vi "FOS_CL_run.vi"() -> ()   [LabVIEW 2019]
uses:
  <vilib>/myRIO/Instrument Drivers/Onboard IO/DIO/typedefs/DIO Reference.ctl
  <vilib>/myRIO/Common/Instrument Driver Framework/Utilities/typedefs/myRIO Generic Hardware Reference.ctl
  <vilib>/myRIO/Common/Instrument Driver Framework/Utilities/typedefs/Hardware Version Enum.ctl
  <vilib>/myRIO/Common/Instrument Driver Framework/Utilities/typedefs/myRIO v1.0 Reference.ctl
  <vilib>/myRIO/Common/Instrument Driver Framework/Utilities/typedefs/Generic FPGA Reference.ctl
  <vilib>/myRIO/Common/Instrument Driver Framework/myRIO v1.0/DIO/typedefs/DIO Channels List.ctl
  <vilib>/myRIO/Common/Instrument Driver Framework/myRIO v1.0/DIO/typedefs/DIO Channels Enum.ctl
  <vilib>/userDefined/High Color/nirio_resource_hc.ctl
  <vilib>/myRIO/Instrument Drivers/Onboard IO/SPI/typedefs/SPI User Configuration.ctl
  <vilib>/myRIO/Common/Instrument Driver Framework/myRIO v1.0/SPI/typedefs/SPI Clock Phase.ctl
  <vilib>/myRIO/Common/Instrument Driver Framework/myRIO v1.0/SPI/typedefs/SPI Clock Polarity.ctl
  <vilib>/myRIO/Common/Instrument Driver Framework/myRIO v1.0/SPI/typedefs/SPI Data Direction.ctl
  <vilib>/myRIO/Common/Instrument Driver Framework/myRIO v1.0/SPI/typedefs/SPI Frame Length.ctl
  <vilib>/myRIO/Instrument Drivers/Onboard IO/SPI/typedefs/SPI Reference.ctl
  <vilib>/myRIO/Common/Instrument Driver Framework/myRIO v1.0/SPI/typedefs/SPI Channels Enum.ctl
  <vilib>/myRIO/Instrument Drivers/Onboard IO/SPI/typedefs/SPI Configuration.ctl
  <vilib>/Platform/TimedLoop/XDataNode/timing_clust.ctl
  <vilib>/Platform/TimedLoop/XDataNode/nitl_modes.ctl
  <vilib>/Platform/TimedLoop/XDataNode/wakeup.ctl
  <vilib>/myRIO/Instrument Drivers/Onboard IO/AI/typedefs/AI Reference.ctl
  <vilib>/myRIO/Common/Instrument Driver Framework/myRIO v1.0/AI/typedefs/AI Channels List.ctl
  <vilib>/myRIO/Common/Instrument Driver Framework/myRIO v1.0/AI/typedefs/AI Channels Enum.ctl
  <vilib>/myRIO/Common/Instrument Driver Framework/Utilities/typedefs/Analog Scaling Constants List.ctl
  <vilib>/myRIO/Common/Instrument Driver Framework/Utilities/typedefs/Analog Scaling Constants.ctl
  <vilib>/myRIO/Common/Instrument Driver Framework/Utilities/vis/Is FPGA Ref Available.vi
  <vilib>/myRIO/Common/Instrument Driver Framework/myRIO v1.0/DIO/vis/myRIO v1.1 Open DIO.vi
  <vilib>/myRIO/Instrument Drivers/Onboard IO/DIO/vis/Write.vi
  <vilib>/myRIO/Common/Instrument Driver Framework/myRIO v1.0/SPI/vis/myRIO v1.1 Open SPI.vi
  <vilib>/myRIO/Instrument Drivers/Onboard IO/SPI/vis/Configure.vi
  <vilib>/myRIO/Instrument Drivers/Onboard IO/SPI/vis/Write Read.vi
  <vilib>/myRIO/Common/Instrument Driver Framework/myRIO v1.0/AI/vis/myRIO v1.1 Open AI.vi
  <vilib>/myRIO/Instrument Drivers/Onboard IO/AI/vis/Read.vi
  <vilib>/myRIO/Common/Instrument Driver Framework/Utilities/vis/Validate Channels.vi
  <vilib>/myRIO/Common/Instrument Driver Framework/myRIO v1.0/DIO/vis/myRIO v1.0 Reserve DIO.vi
  <vilib>/myRIO/Common/Instrument Driver Framework/myRIO v1.0/SPI/vis/myRIO v1.0 Reserve SPI.vi
  <vilib>/myRIO/Common/Instrument Driver Framework/myRIO v1.0/AI/vis/myRIO v1.0 Reserve AI.vi
  <vilib>/myRIO/Common/Instrument Driver Framework/myRIO v1.0/Resource Manager/vis/myRIO v1.0 Reserve Channel List.vi
  <vilib>/myRIO/Common/Instrument Driver Framework/myRIO v1.0/DIO/vis/myRIO v1.0 Build MUX Configuration DIO.vi
  <vilib>/myRIO/Common/Instrument Driver Framework/myRIO v1.0/SPI/vis/myRIO v1.0 Build MUX Configuration SPI.vi
  <vilib>/myRIO/Common/Instrument Driver Framework/myRIO v1.0/AI/vis/myRIO v1.0 Build MUX Configuration AI.vi
  <vilib>/myRIO/Common/Instrument Driver Framework/myRIO v1.0/Resource Manager/vis/myRIO v1.0 Reserve Channel.vi
  <vilib>/myRIO/Common/Instrument Driver Framework/myRIO v1.0/Resource Manager/vis/myRIO v1.0 Unreserve Channel.vi
  <vilib>/myRIO/Common/Instrument Driver Framework/myRIO v1.0/Resource Manager/vis/myRIO v1.0 Create Configuration List.vi
  <vilib>/myRIO/Common/Instrument Driver Framework/myRIO v1.0/Resource Manager/vis/myRIO v1.0 Build Mutex Name.vi
  <vilib>/Utility/VariantDataType/GetNumericInfo.vi
  <vilib>/Utility/error.llb/Error Cluster From Error Code.vi
  <vilib>/myRIO/Common/Instrument Driver Framework/myRIO v1.0/myRIO v1.1 Open.vi
  <vilib>/myRIO/Common/Instrument Driver Framework/Utilities/vis/IO Manager.vi
  <vilib>/myRIO/Common/Instrument Driver Framework/Utilities/vis/Configuration Manager.vi
  <vilib>/myRIO/Common/Instrument Driver Framework/myRIO v1.0/Resource Manager/vis/myRIO v1.0 Configure IO.vi
  <vilib>/myRIO/Common/Instrument Driver Framework/myRIO v1.0/myRIO v1.0 Close.vi
  <vilib>/myRIO/Common/Instrument Driver Framework/myRIO v1.0/DIO/vis/myRIO v1.0 Write DIO.vi
  Global_vars.vi
  <vilib>/myRIO/Common/Instrument Driver Framework/myRIO v1.0/SPI/vis/myRIO v1.0 Configure SPI.vi
  <vilib>/myRIO/Common/Instrument Driver Framework/myRIO v1.0/SPI/vis/myRIO v1.0 Write Read SPI.vi
  <vilib>/Utility/file.llb/Read Delimited Spreadsheet (DBL).vi
  <vilib>/Utility/file.llb/Write Delimited Spreadsheet (DBL).vi
  <vilib>/myRIO/Common/Instrument Driver Framework/myRIO v1.0/AI/vis/myRIO v1.0 Get Scaling Constants AI.vi
  <vilib>/myRIO/Common/Instrument Driver Framework/myRIO v1.0/AI/vis/myRIO v1.0 Read AI.vi
  <vilib>/addons/control/pid/pid.llb/PID (DBL).vi
  <vilib>/myRIO/Express VI/Onboard IO/DO/DO Express VI.xnode
  <vilib>/myRIO/Instrument Drivers/Onboard IO/DIO/vis/myRIO DIO Open.xnode
  <vilib>/myRIO/Express VI/Onboard IO/SPI/SPI Express VI.xnode
  <vilib>/myRIO/Instrument Drivers/Onboard IO/SPI/vis/myRIO SPI Open.xnode
  <vilib>/Platform/TimedLoop/XDataNode/XDataNode.xnode
  <vilib>/myRIO/Express VI/Onboard IO/AI/AI Express VI.xnode
  <vilib>/myRIO/Instrument Drivers/Onboard IO/AI/vis/myRIO AI Open.xnode
  <vilib>/Platform/TimedLoop/XDataNode/XDNodeRunTimeDep.lvlib
  <vilib>/ptbypt/NI_PtbyPt.lvlib
  <vilib>/addons/control/pid/NI_PID_pid.lvlib
  <vilib>/myRIO/Instrument Drivers/Onboard IO/DIO/DIO.lvlib
  <vilib>/myRIO/Instrument Drivers/Onboard IO/SPI/SPI.lvlib
  <vilib>/myRIO/Instrument Drivers/Onboard IO/AI/AI.lvlib
panel:
  out "yk":dbl(graph)
  out "Control signals":T1(graph)
  in  "Model off on":bool
  out "forceInd":dbl
  out "controlVariable":dbl[](graph)
  out "controlSignal":dbl[](graph)
  out "Control signal":dbl(graph)
  in  "stop test":bool
  in  "stop":bool
  in  "Mode test CL":bool
  out "rawF":dbl[](graph)
  out "Control performance":cluster{"F ref":dbl, "raw F":dbl}(graph)
  in  "File path":path=path "C:/Opto/fatigue_plantar2.txt"
  out "Fref":dbl[](graph)
  in  "Setup":T2(tab)
  in  "Sin Sq":bool
  in  "Ref freq (Hz)":dbl
  in  "Ref amp (mN)":dbl
  in  "Offset (mN)":dbl
  in  "output range":cluster{"output high":dbl, "output low":dbl}={"output high"=100.0, "output low"=-100.0} {"output low" format="%.2f"; "output high" format="%.2f"}
  in  "PID gains":T3={"proportional gain (Kc)"=1.0, "integral time (Ti, min)"=0.01, "derivative time (Td, min)"=0.0} {"derivative time (Td, min)" format="%.3f"; "integral time (Ti, min)" format="%.3f"; "proportional gain (Kc)" format="%.3f"}
  in  "Gyk":dbl
  in  "maxCS":dbl
  in  "minCS":dbl
  in  "Gff":dbl
  in  "y3":dbl
  in  "y2":dbl
  in  "y1":dbl
  in  "x0":dbl
  in  "x1":dbl
  in  "x2":dbl
  in  "x3":dbl
  in  "Offset2 (mN)":dbl
  in  "delta force (mN)":dbl
  in  "PW test (0-100%)":dbl
  in  "Stim Frequency (Hz)":dbl=39.0
  in  "Ampitude (0<x<100%)":dbl=0.05
  out "Val to dig pot":u8
  in  "SPI command (0x12)":u8 format="%x"
  out "feedforward missed":dbl
  out "controller missed":dbl
  out "stim missed":dbl
  out "force reading missed":dbl
  out "save missed":dbl
  out "ref missed":dbl
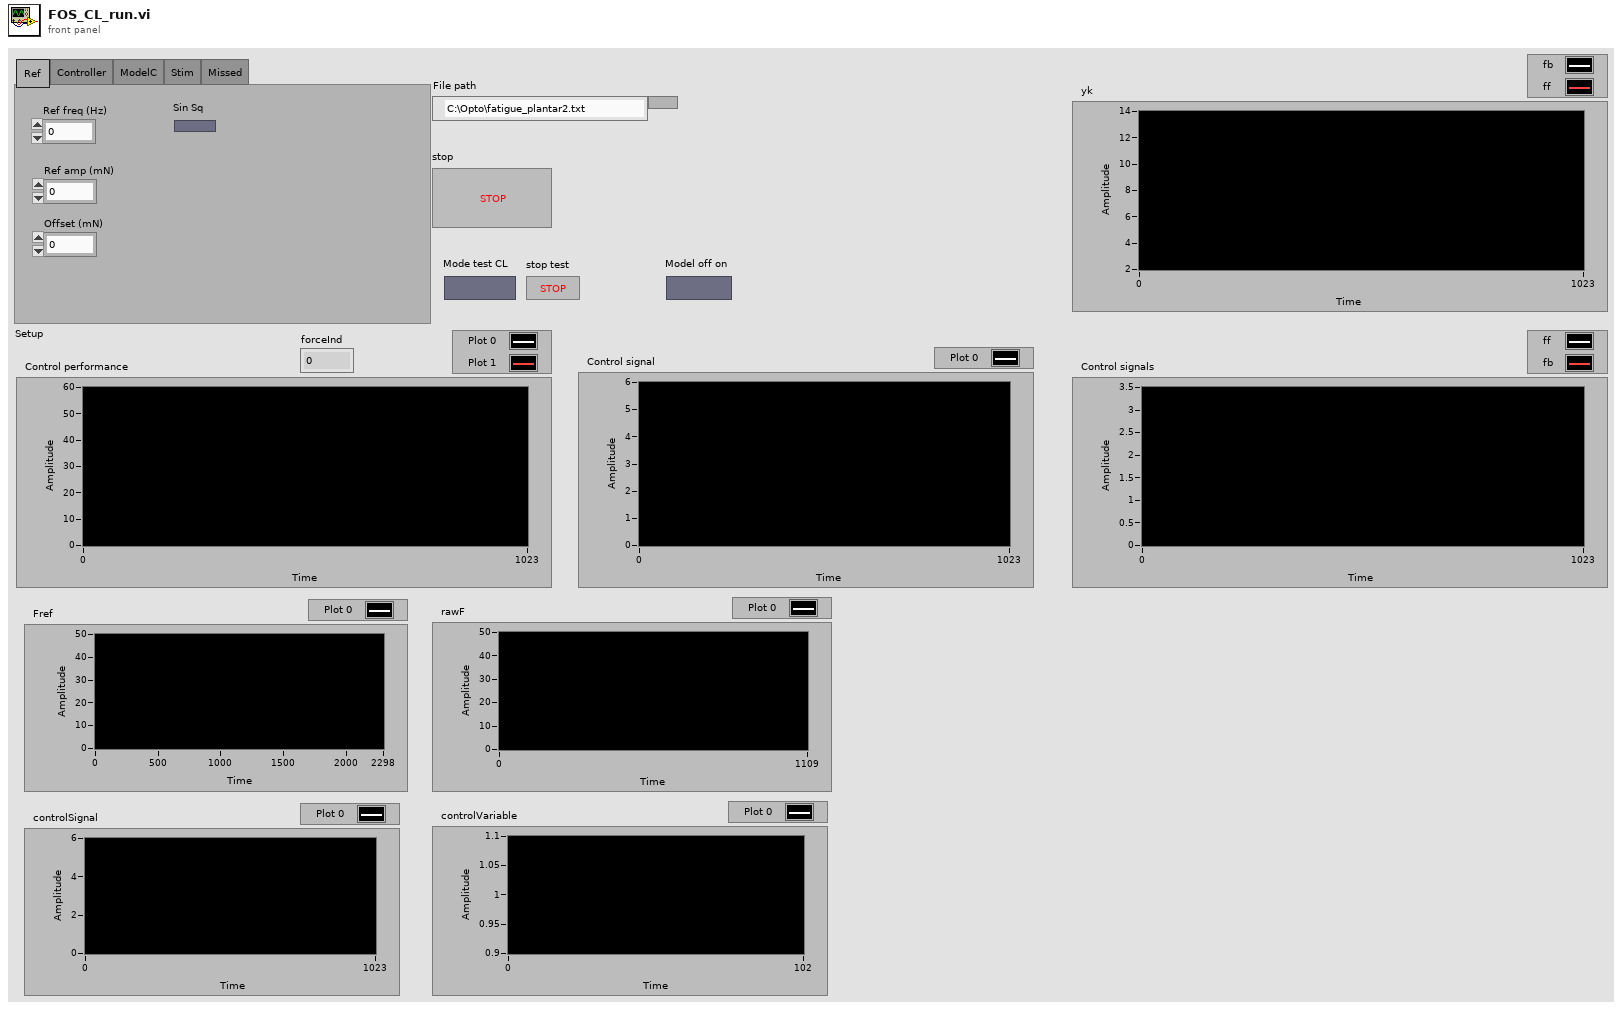
[diagram p1: front panel]
types:
  T1 = cluster{"control signal ff":dbl, "control signal fb":dbl}
  T2 = enum32{"Ref ", "Controller", "ModelC", "Stim", "Missed"}
  T3 = cluster{"proportional gain (Kc)":dbl, "integral time (Ti, min)":dbl, "derivative time (Td, min)":dbl}
  T4 = typedef "DIO.lvlib/DIO Reference.ctl" = cluster{"myRIO Reference":T5, "DIO Channels List":T9}
  T5 = typedef "myRIO Generic Hardware Reference.ctl" = cluster{"myRIO Model":T6, "myRIO Hardware Reference":T7}
  T6 = typedef "Hardware Version Enum.ctl" = enum16{"Unknown", "myRIO-1900", "myRIO-1950", "roboRIO", "NI ELVIS RIO CM", "ELVIS III"}
  T7 = typedef "myRIO v1.0 Reference.ctl" = cluster{"Generic FPGA Reference":T8, "Allow multiple opens":bool}
  T8 = typedef "Generic FPGA Reference.ctl" = refnum<k20>
  T9 = typedef "DIO Channels List.ctl" = T10[]
  T10 = typedef "DIO Channels Enum.ctl" = enum16{"Not Connected", "C/DIO0", "C/DIO1", "C/DIO2", "C/DIO3", "C/DIO4", "C/DIO5", "C/DIO6", "C/DIO7", "A/DIO0", "A/DIO1", "A/DIO2", "A/DIO3", "A/DIO4", "A/DIO5", "A/DIO6", "A/DIO7", "A/DIO8", "A/DIO9", "A/DIO10", "A/DIO11", "A/DIO12", "A/DIO13", "A/DIO14", "A/DIO15", "A/DIO16", "A/DIO17", "A/DIO18", "A/DIO19", "B/DIO0", "B/DIO1", "B/DIO2", "B/DIO3", "B/DIO4", "B/DIO5", "B/DIO6", "B/DIO7", "B/DIO8", "B/DIO9", "B/DIO10", "B/DIO11", "B/DIO12", "B/DIO13", "B/DIO14", "B/DIO15", "B/DIO16", "B/DIO17", "B/DIO18", "B/DIO19", "LED0", "LED1", "LED2", "LED3", "Button0", "DIO/DIO0", "DIO/DIO1", "DIO/DIO2", "DIO/DIO3", "DIO/DIO4", "DIO/DIO5", "DIO/DIO6", "DIO/DIO7", "DIO/DIO8", "DIO/DIO9", "SPI/CS0", "SPI/CS1", "SPI/CS2", "SPI/CS3", "LED RADIO (Green)", "LED RADIO (Red)", "LED COMM (Green)", "LED COMM (Red)", "LED MODE (Green)", "LED MODE (Red)"}
  T11 = typedef "nirio_resource_hc.ctl" = tag
  T12 = typedef "SPI.lvlib/SPI Reference.ctl" = cluster{"myRIO Reference":T5, "SPI Channels Enum":T13, "SPI Configuration":T14}
  T13 = typedef "SPI Channels Enum.ctl" = enum16{"Not Connected", "A/SPI", "B/SPI", "SPI/SPI"}
  T14 = typedef "SPI.lvlib/SPI Configuration.ctl" = cluster{"Frequency [Hz]":dbl, "Clock Phase":T15, "Clock Polarity":T16, "Data Direction":T17, "Frame Length":T18}
  T15 = typedef "SPI Clock Phase.ctl" = enum8{"Leading", "Trailing"}
  T16 = typedef "SPI Clock Polarity.ctl" = enum8{"Low", "High"}
  T17 = typedef "SPI Data Direction.ctl" = enum8{"Most significant bit first", "Least significant bit first"}
  T18 = typedef "SPI Frame Length.ctl" = u8
  T19 = typedef "SPI.lvlib/SPI User Configuration.ctl" = cluster{"Frequency [Hz]":dbl, "Clock Phase":T15, "Clock Polarity":T16, "Data Direction":T17, "Frame Length":T18}
  T20 = typedef "XDNodeRunTimeDep.lvlib/timing_clust.ctl" = cluster{"Expected End [f-1]":u64, "Actual End [f-1]":u64, "Finished Late? [f-1]":bool, "Expected End [i-1]":u64, "Actual End [i-1]":u64, "Finished Late? [i-1]":bool, "Expected Start [i]":u64, "Actual Start [i]":u64, "Expected Start [f]":u64, "Actual Start [f]":u64, "Source Name":string, "Structure Name":string, "Period":i64, "Deadline":i64, "Offset":i64, "Start":i64, "Priority":i32, "Timeout":i32, "Mode":T21, "Wakeup Reason":T22, "Error":errorcluster, "Source Type":string, "Secondary Source Type":string, "Global End Time":u64, "Global Start Time":u64, "Frame Duration":u64, "Iteration Duration":u64, "Assigned CPU":i32, "I/O Scan Engine Mode":u32}
  T21 = typedef "XDNodeRunTimeDep.lvlib/nitl_modes.ctl" = enum32{"No Change", "Process missed periods, maintain original phase", "Discard missed periods, maintain original phase", "Process missed periods, ignore original phase", "Discard missed periods, ignore original phase"}
  T22 = typedef "XDNodeRunTimeDep.lvlib/wakeup.ctl" = enum32{"Normal", "Aborted", "Asynchronous wakeup", "Timing source error", "Timed loop error", "Timeout"}
  T23 = typedef "AI.lvlib/AI Reference.ctl" = cluster{"myRIO Reference":T5, "AI Channels List":T24, "AI Scaling Constants List":T26}
  T24 = typedef "AI Channels List.ctl" = T25[]
  T25 = typedef "AI Channels Enum.ctl" = enum16{"Not Connected", "AudioIn/Left", "AudioIn/Right", "C/AI0", "C/AI1", "A/AI0", "A/AI1", "A/AI2", "A/AI3", "A/AI4", "A/AI5", "A/AI6", "A/AI7", "B/AI0", "B/AI1", "B/AI2", "B/AI3", "B/AI4", "B/AI5", "B/AI6", "B/AI7", "AI/AI0", "AI/AI1", "AI/AI2", "AI/AI3", "A/AI0 (DIFF)", "A/AI1 (DIFF)", "A/AI2 (DIFF)", "A/AI3 (DIFF)", "B/AI0 (DIFF)", "B/AI1 (DIFF)", "B/AI2 (DIFF)", "B/AI3 (DIFF)"}
  T26 = typedef "Analog Scaling Constants List.ctl" = T27[]
  T27 = typedef "Analog Scaling Constants.ctl" = cluster{"LSB Weight (Volts)":dbl, "Offset (Volts)":dbl, "Signed?":bool}
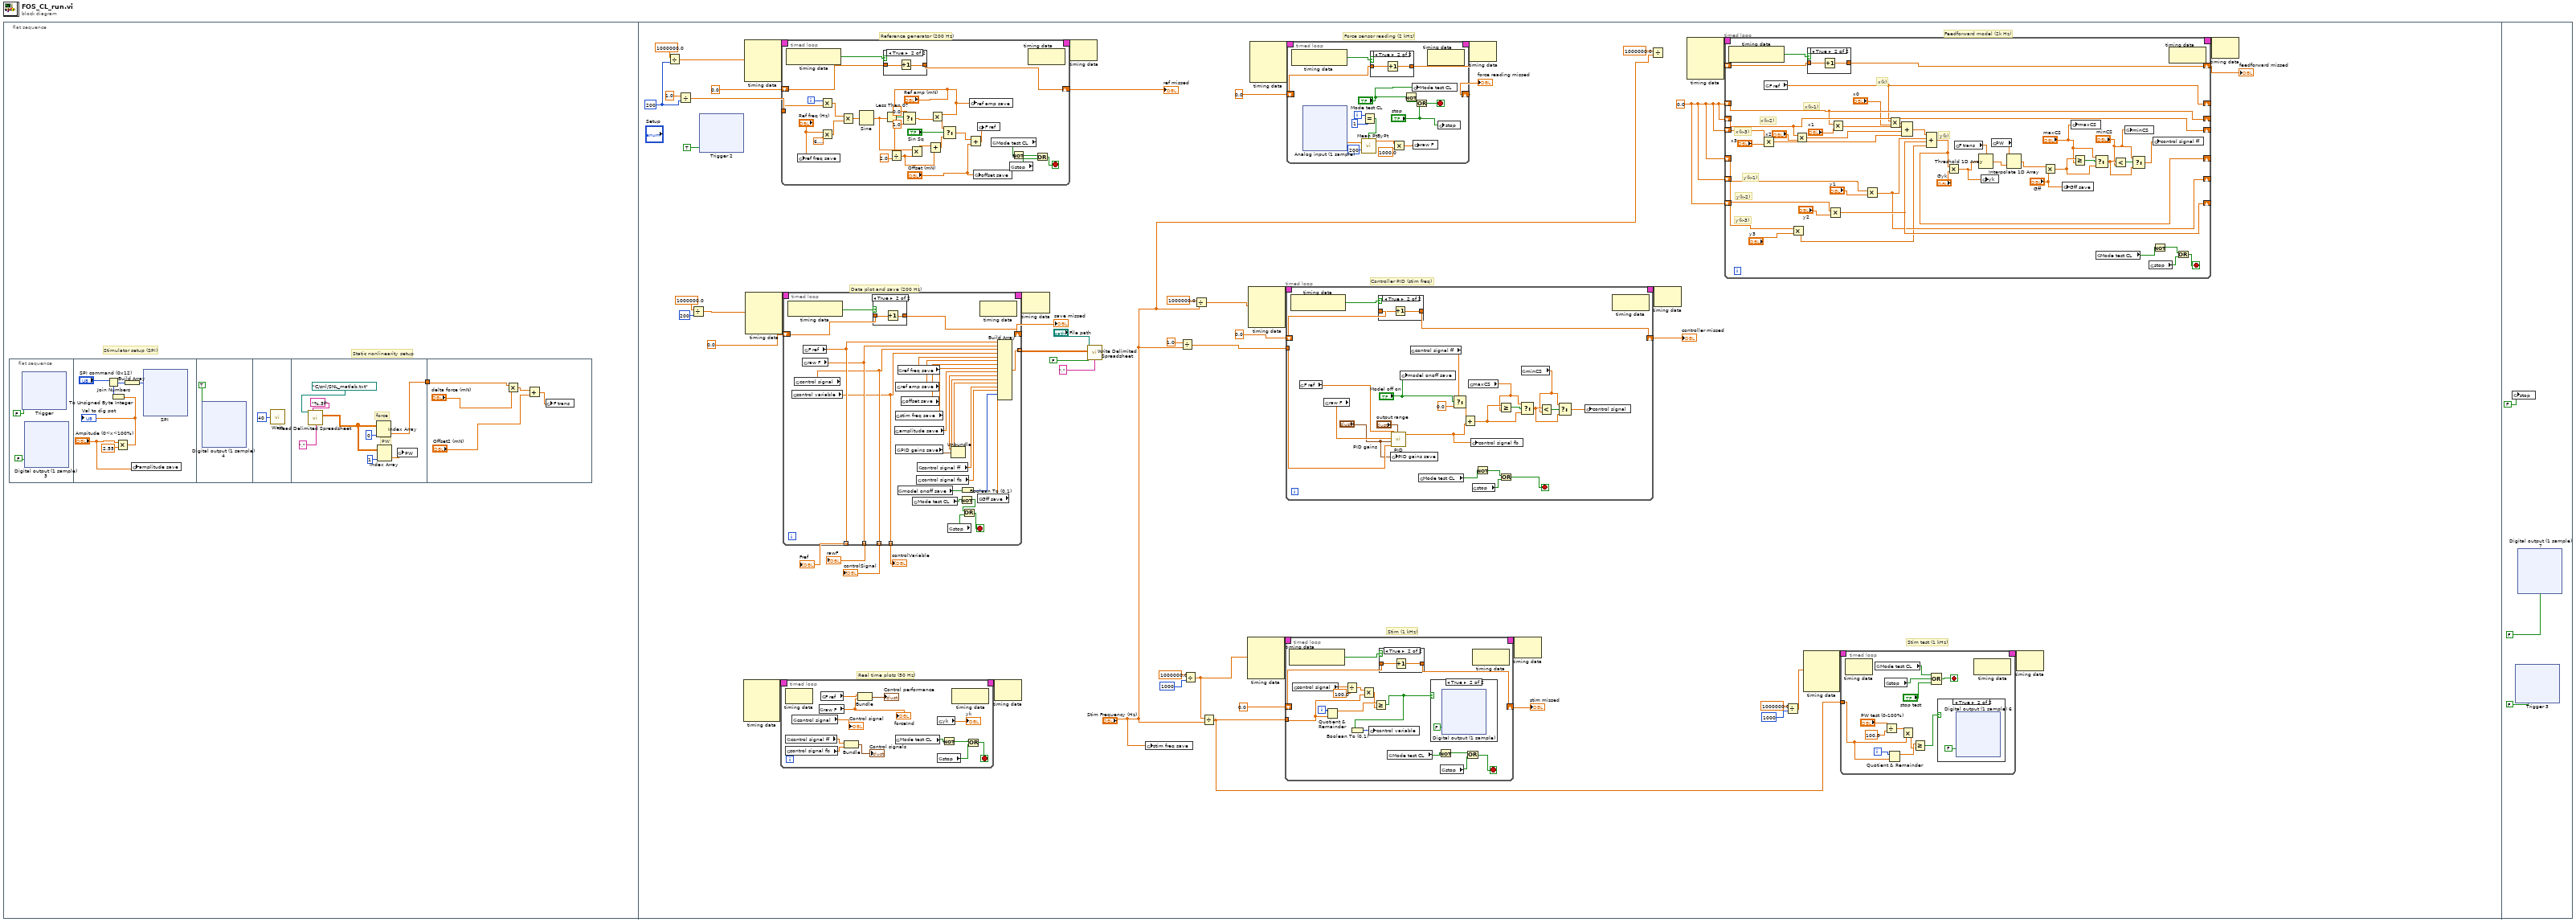
[diagram p0: block diagram]
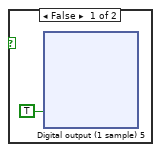
[diagram p3: hidden frame]
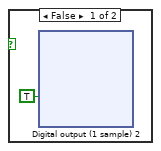
[diagram p5: hidden frame]
diagram:
  n1 = flat-sequence {
    frame #0 {
      # "Static nonlinearity setup"
      # "Stimulator setup (SPI)"
      n2 = flat-sequence {
        tunnel: [w156] -> w1
        tunnel: w1 -> [w167]
        frame #0 {
          n3 = xnode "Trigger"("C/DIO7 (DIO7)"=FALSE) -> ()  [unwired: 1 in, 1 out]
          n4 = xnode "Digital output (1 sample) 3"("CS (A/DIO4 (Pin 19))"=FALSE ("CS (B/DIO4 (Pin 19))")) -> ()  [unwired: 1 in, 1 out]
        }
        frame #1 {
          n5 = Multiply(x="Ampitude (0<x<100%)", y=2.55) -> (x*y=w80:dbl)
          "Val to dig pot" <- w80
          n6 = To Unsigned Byte Integer(number=w80) -> (unsigned 8bit integer=w79:u8)
          n7 = Join Numbers(hi="SPI command (0x12)", lo=w79) -> ((hi.lo)=w77:u16)
          n8 = Build Array(w77) -> (w78:u16[])
          n9 = global write "Global_vars.vi" "amplitude save"("Ampitude (0<x<100%)") -> ()
          n10 = xnode "SPI"("Frames to Write"=w78) -> ()  [unwired: 1 in, 2 out]
        }
        frame #2 {
          n11 = xnode "Digital output (1 sample) 4"("CS (A/DIO4 (Pin 19))"=TRUE ("CS (B/DIO4 (Pin 19))")) -> ()  [unwired: 1 in, 1 out]
        }
        frame #3 {
          n12 = call "Wait"("Count(uSec)"=u32 40) -> ()  [unwired: 1 out]
        }
        frame #4 {
          # "PW"
          # "force"
          n13 = call-poly <vilib>:"Read Delimited Spreadsheet.vi"("file path (dialog if empty)"=path "C:/snl/SNL_matlab.txt", "format (%.3f)"="%.3f", "delimiter (\\t)"="," ("delimiter (\\t)")) -> ("all rows"=w162:dbl[][])  [unwired: 7 in, 5 out]
          n14 = Index Array(array=w162, index (col)=0 ("disabled index (col)")) -> (element=w156:dbl[])  [unwired: 1 in]
          n15 = Index Array(array=w162, index (col)=1 ("disabled index (col)")) -> (element=w163:dbl[])  [unwired: 1 in]
          n16 = global write "Global_vars.vi" "PW"(w163) -> ()
        }
        frame #5 {
          n17 = Multiply(x=w167, y="delta force (mN)") -> (x*y=w168:dbl[])
          n18 = Add(x=w168, y="Offset2 (mN)") -> (x+y=w166:dbl[])
          n19 = global write "Global_vars.vi" "F trans"(w166) -> ()
        }
      }
    }
    frame #1 {
      w173 = 0.0 ("F ref")
      w218 = 200
      # "Feedforward model (2k Hz)"
      # "Stim test (1 kHz)"
      # "Stim (1 kHz)"
      # "Controller PID (stim freq)"
      # "Force sensor reading (2 kHz)"
      # "Real time plots (50 Hz)"
      # "Data plot and save (200 Hz)"
      # "Reference generator (200 Hz)"
      n20 = Divide(x=1000000.0, y=w218) -> (x/y=w220:dbl)
      n21 = Divide(x=1.0, y=w218) -> (x/y=w223:dbl)
      n22 = Divide(x=1000000.0, y=200) -> (x/y=w217:dbl)
      n23 = xnode "Trigger 2"("C/DIO7 (DIO7)"=TRUE) -> ()  [unwired: 1 in, 1 out]
      n24 = node-c288() -> (w210:T20)  [unwired: 4 in]
      n25 = node-c288(w220) -> (w226:T20)  [unwired: 3 in]
      n26 = node-c288(w217) -> (w222:T20)  [unwired: 3 in]
      n27 = timed-loop {
        timing: w210 -> [_]
        timing-out: [_] -> w209
        stop <- w604 stop-if-true
        n28 = node-c288() -> ()  [unwired: 1 in, 1 out]
        n29 = global read "Global_vars.vi" "control signal fb"() -> (w598:dbl)
        n30 = global read "Global_vars.vi" "control signal ff"() -> (w599:dbl)
        n31 = global read "Global_vars.vi" "control signal"() -> (→"Control signal":dbl)
        n32 = global read "Global_vars.vi" "raw F"() -> (w600:dbl)
        "forceInd" <- w600
        n33 = global read "Global_vars.vi" "F ref"() -> (w601:dbl)
        n34 = Bundle("control signal ff"=w599, "control signal fb"=w598) -> (→"Control signals":T1)  [unwired: 1 in]
        n35 = Bundle("F ref"=w601, "raw F"=w600) -> (→"Control performance":cluster{"F ref":dbl, "raw F":dbl})  [unwired: 1 in]
        n36 = global read "Global_vars.vi" "Mode test CL"() -> (w607:bool)
        n37 = global read "Global_vars.vi" "yk"() -> (→"yk":dbl)
        n38 = global read "Global_vars.vi" "stop"() -> (w605:bool)
        n39 = Not(x=w607) -> (.not. x?=w606:bool)
        n40 = node-c288() -> ()  [unwired: 1 in, 1 out]
        n41 = Or(x=w606, y=w605) -> (x .or. y?=w604:bool)
      }
      n42 = timed-loop {
        timing: w226 -> [_]
        timing-out: [_] -> w225
        tunnel: w223 -> [w674]
        shift-right: [w655] -> w207
        shift-left: 0.0 -> [w656]
        i -> [w675]
        stop <- w654 stop-if-true
        n43 = node-c288() -> (w657:bool)  [unwired: 1 in]
        n44 = global write "Global_vars.vi" "ref freq save"("Ref freq (Hz)") -> ()
        n45 = Multiply(x=w675, y=w674) -> (x*y=w673:dbl)
        n46 = Multiply(x="Ref freq (Hz)", y=6.283185307179586) -> (x*y=w672:dbl)
        n47 = Multiply(x=w673, y=w672) -> (x*y=w671:dbl)
        n48 = Sine(x=w671) -> (sin(x)=w662:dbl)
        n49 = case shown="True" w657 {
          tunnel: w656 -> [w677 w679]
          tunnel: [w677 w678] -> w655
          frame False {
          }
          frame True {
            n50 = Increment(x=w679) -> (x+1=w678:dbl)
          }
        }
        n51 = Less Than 0?(x=w662) -> (x < 0?=w670:bool)
        n52 = Divide(x="Ref amp (mN)", y=2.0) -> (x/y=w661:dbl)
        n53 = Select(t=0.0, s=w670, f=1.0) -> (s? t:f=w665:dbl)
        n54 = Multiply(x=w662, y=w661) -> (x*y=w660:dbl)
        n55 = Add(x=w660, y=w661) -> (x+y=w659:dbl)
        n56 = Multiply(x="Ref amp (mN)", y=w665) -> (x*y=w664:dbl)
        n57 = Select(t=w664, s="Sin Sq", f=w659) -> (s? t:f=w658:dbl)
        n58 = Add(x=w658, y="Offset (mN)") -> (x+y=w666:dbl)
        n59 = global write "Global_vars.vi" "ref amp save"("Ref amp (mN)") -> ()
        n60 = global write "Global_vars.vi" "offset save"("Offset (mN)") -> ()
        n61 = global write "Global_vars.vi" "F ref"(w666) -> ()
        n62 = global read "Global_vars.vi" "Mode test CL"() -> (w652:bool)
        n63 = global read "Global_vars.vi" "stop"() -> (w653:bool)
        n64 = Not(x=w652) -> (.not. x?=w651:bool)
        n65 = node-c288() -> ()  [unwired: 1 in, 1 out]
        n66 = Or(x=w651, y=w653) -> (x .or. y?=w654:bool)
      }
      "ref missed" <- w207
      n67 = timed-loop {
        timing: w222 -> [_]
        timing-out: [_] -> w221
        tunnel: [w634] -> w213 mode=indexing
        shift-right: [w635] -> w205
        shift-left: 0.0 -> [w636]
        tunnel: [w633] -> w186 mode=indexing
        tunnel: [w632] -> w185 mode=indexing
        tunnel: [w627] -> w178 mode=indexing
        tunnel: [w626] -> w177 mode=indexing
        stop <- w630 stop-if-true
        n68 = node-c288() -> (w637:bool)  [unwired: 1 in]
        n69 = global read "Global_vars.vi" "control variable"() -> (w626:dbl)
        n70 = global read "Global_vars.vi" "control signal"() -> (w627:dbl)
        n71 = global read "Global_vars.vi" "raw F"() -> (w633:dbl)
        n72 = global read "Global_vars.vi" "F ref"() -> (w634:dbl)
        n73 = case shown="True" w637 {
          tunnel: w636 -> [w638 w640]
          tunnel: [w638 w639] -> w635
          frame False {
          }
          frame True {
            n74 = Increment(x=w640) -> (x+1=w639:dbl)
          }
        }
        n75 = global read "Global_vars.vi" "amplitude save"() -> (w621:dbl)
        n76 = global read "Global_vars.vi" "stim freq save"() -> (w622:dbl)
        n77 = global read "Global_vars.vi" "ref amp save"() -> (w624:dbl)
        n78 = global read "Global_vars.vi" "PID gains save"() -> (w620:T3)
        n79 = global read "Global_vars.vi" "ref freq save"() -> (w625:dbl)
        n80 = global read "Global_vars.vi" "model onoff save"() -> (w614:bool)
        n81 = global read "Global_vars.vi" "offset save"() -> (w623:dbl)
        n82 = global read "Global_vars.vi" "Mode test CL"() -> (w628:bool)
        n83 = global read "Global_vars.vi" "control signal fb"() -> (w615:dbl)
        n84 = global read "Global_vars.vi" "control signal ff"() -> (w616:dbl)
        n85 = global read "Global_vars.vi" "stop"() -> (w631:bool)
        n86 = Unbundle(w620) -> ("proportional gain (Kc)"=w619:dbl, "integral time (Ti, min)"=w618:dbl, "derivative time (Td, min)"=w617:dbl)
        n87 = Not(x=w628) -> (.not. x?=w629:bool)
        n88 = Boolean To (0,1)(Boolean=w614) -> (0, 1=w613:i16)
        n89 = Or(x=w629, y=w631) -> (x .or. y?=w630:bool)
        n90 = global read "Global_vars.vi" "Gff save"() -> (w612:dbl)
        n91 = node-c288() -> ()  [unwired: 1 in, 1 out]
        n92 = Build Array(w634, w633, w627, w626, w625, w624, w623, w622, w621, w619, w618, w617, w616, w615, w613, w612) -> (w632:dbl[])
      }
      "Fref" <- w213
      "save missed" <- w205
      "rawF" <- w186
      "controlSignal" <- w178
      "controlVariable" <- w177
      n93 = node-c288(w209) -> ()  [unwired: 1 out]
      n94 = node-c288(w221) -> ()  [unwired: 1 out]
      n95 = node-c288(w225) -> ()  [unwired: 1 out]
      n96 = call-poly <vilib>:"Write Delimited Spreadsheet.vi"("file path (dialog if empty)"="File path", "2D data"=w185, "append to file? (new file:F)"=FALSE, "delimiter (\\t)"="," ("delimiter (\\t)")) -> ()  [unwired: 10 in, 2 out]
      n97 = global write "Global_vars.vi" "stim freq save"("Stim Frequency (Hz)") -> ()
      n98 = Divide(x=1.0, y="Stim Frequency (Hz)") -> (x/y=w189:dbl)
      n99 = Divide(x=1000000.0, y=1000) -> (x/y=w194:dbl)
      n100 = Divide(x=1000000.0, y="Stim Frequency (Hz)") -> (x/y=w169:dbl)
      n101 = Divide(x=w194, y="Stim Frequency (Hz)") -> (x/y=w179:dbl)
      n102 = node-c288(w194) -> (w198:T20)  [unwired: 3 in]
      n103 = node-c288(w169) -> (w200:T20)  [unwired: 3 in]
      n104 = node-c288() -> (w204:T20)  [unwired: 4 in]
      n105 = timed-loop {
        timing: w198 -> [_]
        timing-out: [_] -> w197
        tunnel: w179 -> [w416]
        shift-right: [w413] -> w192
        shift-left: 0.0 -> [w414]
        i -> [w415]
        stop <- w407 stop-if-true
        n106 = node-c288() -> (w412:bool)  [unwired: 1 in]
        n107 = global read "Global_vars.vi" "control signal"() -> (w419:dbl)
        n108 = Quotient & Remainder(x=w415, y=w416) -> (x-y*floor(x/y)=w405:dbl)  [unwired: 1 out]
        n109 = Divide(x=w419, y=100.0) -> (x/y=w417:dbl)
        n110 = Multiply(x=w417, y=w416) -> (x*y=w404:dbl)
        n111 = Greater Or Equal?(x=w405, y=w404) -> (x >= y?=w411:bool)
        n112 = Boolean To (0,1)(Boolean=w411) -> (0, 1=w410:i16)
        n113 = global write "Global_vars.vi" "control variable"(w410) -> ()
        n114 = case shown="True" w412 {
          tunnel: w414 -> [w420 w422]
          tunnel: [w420 w421] -> w413
          frame False {
          }
          frame True {
            n115 = Increment(x=w422) -> (x+1=w421:dbl)
          }
        }
        n116 = global read "Global_vars.vi" "Mode test CL"() -> (w406:bool)
        n117 = case shown="True" w411 {
          frame False {
            n118 = xnode "Digital output (1 sample) 2"("CH1 (A/DIO8 (Pin 27))"=TRUE) -> ()  [unwired: 1 in, 1 out]
          }
          frame True {
            n119 = xnode "Digital output (1 sample)"("CH1 (A/DIO8 (Pin 27))"=FALSE) -> ()  [unwired: 1 in, 1 out]
          }
        }
        n120 = Not(x=w406) -> (.not. x?=w408:bool)
        n121 = global read "Global_vars.vi" "stop"() -> (w409:bool)
        n122 = Or(x=w408, y=w409) -> (x .or. y?=w407:bool)
        n123 = node-c288() -> ()  [unwired: 1 in, 1 out]
      }
      "stim missed" <- w192
      n124 = timed-loop {
        timing: w200 -> [_]
        timing-out: [_] -> w199
        tunnel: w189 -> [w523]
        shift-right: [w520] -> w187
        shift-left: 0.0 -> [w521]
        stop <- w517 stop-if-true
        n125 = node-c288() -> (w522:bool)  [unwired: 1 in]
        n126 = global read "Global_vars.vi" "F ref"() -> (w512:dbl)
        n127 = global read "Global_vars.vi" "raw F"() -> (w524:dbl)
        n128 = case shown="True" w522 {
          tunnel: w521 -> [w526 w528]
          tunnel: [w526 w527] -> w520
          frame False {
          }
          frame True {
            n129 = Increment(x=w528) -> (x+1=w527:dbl)
          }
        }
        n130 = global write "Global_vars.vi" "PID gains save"("PID gains") -> ()
        n131 = call-poly <vilib>:"PID.vi"("output range"="output range", "dt (s)"=w523, "PID gains"="PID gains", "process variable"=w524, "setpoint"=w512) -> ("output"=w510:dbl)  [unwired: 5 in, 1 out]
        n132 = global write "Global_vars.vi" "model onoff save"("Model off on") -> ()
        n133 = global read "Global_vars.vi" "control signal ff"() -> (w511:dbl)
        n134 = global read "Global_vars.vi" "Mode test CL"() -> (w516:bool)
        n135 = Select(t=w511, s="Model off on", f=0.0) -> (s? t:f=w513:dbl)
        n136 = Add(x=w513, y=w510) -> (x+y=w504:dbl)
        n137 = global read "Global_vars.vi" "maxCS"() -> (w503:dbl)
        n138 = global write "Global_vars.vi" "control signal fb"(w510) -> ()
        n139 = global read "Global_vars.vi" "stop"() -> (w519:bool)
        n140 = Not(x=w516) -> (.not. x?=w518:bool)
        n141 = Greater Or Equal?(x=w504, y=w503) -> (x >= y?=w508:bool)
        n142 = Or(x=w518, y=w519) -> (x .or. y?=w517:bool)
        n143 = Select(t=w503, s=w508, f=w504) -> (s? t:f=w506:dbl)
        n144 = global read "Global_vars.vi" "minCS"() -> (w502:dbl)
        n145 = Less?(x=w506, y=w502) -> (x < y?=w507:bool)
        n146 = Select(t=w502, s=w507, f=w506) -> (s? t:f=w505:dbl)
        n147 = global write "Global_vars.vi" "control signal"(w505) -> ()
        n148 = node-c288() -> ()  [unwired: 1 in, 1 out]
      }
      "controller missed" <- w187
      n149 = timed-loop {
        timing: w204 -> [_]
        timing-out: [_] -> w203
        shift-right: [w544] -> w201
        shift-left: 0.0 -> [w545]
        i -> [w549]
        stop <- w541 stop-if-true
        n150 = node-c288() -> (w546:bool)  [unwired: 1 in]
        n151 = xnode "Analog input (1 sample)"() -> ("C/AI0 (AI0)"=w536:dbl)  [unwired: 1 in, 1 out]
        n152 = Equal?(x=w549, y=1) -> (x = y?=w547:bool)
        n153 = call <vilib>:"Mean PtByPt.vi"("x"=w536, "sample length"=200, "initialize"=w547) -> ("mean"=w538:dbl)  [unwired: 1 in, 1 out]
        n154 = case shown="True" w546 {
          tunnel: w545 -> [w551 w553]
          tunnel: [w551 w552] -> w544
          frame False {
          }
          frame True {
            n155 = Increment(x=w553) -> (x+1=w552:dbl)
          }
        }
        n156 = Multiply(x=w538, y=1000.0) -> (x*y=w537:dbl)
        n157 = Not(x="Mode test CL") -> (.not. x?=w543:bool)
        n158 = global write "Global_vars.vi" "Mode test CL"("Mode test CL") -> ()
        n159 = global write "Global_vars.vi" "raw F"(w537) -> ()
        n160 = Or(x=w543, y="stop") -> (x .or. y?=w541:bool)
        n161 = node-c288() -> ()  [unwired: 1 in, 1 out]
        n162 = global write "Global_vars.vi" "stop"("stop") -> ()
      }
      "force reading missed" <- w201
      n163 = node-c288(w203) -> ()  [unwired: 1 out]
      n164 = node-c288(w197) -> ()  [unwired: 1 out]
      n165 = Divide(x=1000000.0, y="Stim Frequency (Hz)") -> ()  [unwired: 1 out]
      n166 = node-c288(w199) -> ()  [unwired: 1 out]
      n167 = node-c288() -> (w175:T20)  [unwired: 4 in]
      n168 = timed-loop {
        timing: w175 -> [_]
        timing-out: [_] -> w174
        shift-right: [w268] -> w172
        shift-left: _ -> [w269]
        shift-right: [w228] -> _
        shift-left: w173 -> [w243]
        shift-right: [w243] -> _
        shift-left: w173 -> [w245]
        shift-right: [w245] -> _
        shift-left: w173 -> [w248]
        shift-right: [w229] -> _
        shift-left: w173 -> [w256]
        shift-right: [w257] -> _
        shift-left: w173 -> [w262]
        shift-right: [w258] -> _
        shift-left: w173 -> [w261]
        stop <- w264 stop-if-true
        # "y(k)"
        # "y(k-3)"
        # "y(k-2)"
        # "y(k-1)"
        # "x(k-3)"
        # "x(k-2)"
        # "x(k)"
        # "x(k-1)"
        n169 = node-c288() -> (w270:bool)  [unwired: 1 in]
        n170 = Multiply(x=w248, y="x3") -> (x*y=w236:dbl)
        n171 = global read "Global_vars.vi" "F ref"() -> (w228:dbl)
        n172 = Multiply(x=w261, y="y3") -> (x*y=w254:dbl)
        n173 = Multiply(x=w245, y="x2") -> (x*y=w237:dbl)
        n174 = case shown="True" w270 {
          tunnel: w269 -> [w271 w273]
          tunnel: [w271 w272] -> w268
          frame False {
          }
          frame True {
            n175 = Increment(x=w273) -> (x+1=w272:dbl)
          }
        }
        n176 = Multiply(x=w262, y="y2") -> (x*y=w258:dbl)
        n177 = Multiply(x=w243, y="x1") -> (x*y=w238:dbl)
        n178 = Multiply(x=w256, y="y1") -> (x*y=w257:dbl)
        n179 = Multiply(x=w228, y="x0") -> (x*y=w263:dbl)
        n180 = Compound Arithmetic op=ADD(w263, w238, w237, w236) -> (w255:dbl)
        n181 = Compound Arithmetic op=ADD(w255, w257, w258, w254) -> (w229:dbl)
        n182 = Multiply(x=w229, y="Gyk") -> (x*y=w227:dbl)
        n183 = global read "Global_vars.vi" "F trans"() -> (w260:dbl[])
        n184 = Threshold 1D Array(2:w227, 3:w260) -> (0:w253:dbl)  [unwired: 1 in]
        n185 = global write "Global_vars.vi" "yk"(w227) -> ()
        n186 = global read "Global_vars.vi" "PW"() -> (w259:dbl[])
        n187 = Interpolate 1D Array(1:w253, 2:w259) -> (0:w235:dbl)
        n188 = Multiply(x=w235, y="Gff") -> (x*y=w234:dbl)
        n189 = global write "Global_vars.vi" "Gff save"("Gff") -> ()
        n190 = global write "Global_vars.vi" "maxCS"("maxCS") -> ()
        n191 = Greater Or Equal?(x=w234, y="maxCS") -> (x >= y?=w252:bool)
        n192 = Select(t="maxCS", s=w252, f=w234) -> (s? t:f=w250:dbl)
        n193 = global read "Global_vars.vi" "Mode test CL"() -> (w267:bool)
        n194 = Less?(x=w250, y="minCS") -> (x < y?=w251:bool)
        n195 = global write "Global_vars.vi" "minCS"("minCS") -> ()
        n196 = Select(t="minCS", s=w251, f=w250) -> (s? t:f=w249:dbl)
        n197 = global read "Global_vars.vi" "stop"() -> (w265:bool)
        n198 = Not(x=w267) -> (.not. x?=w266:bool)
        n199 = global write "Global_vars.vi" "control signal ff"(w249) -> ()
        n200 = node-c288() -> ()  [unwired: 1 in, 1 out]
        n201 = Or(x=w266, y=w265) -> (x .or. y?=w264:bool)
      }
      "feedforward missed" <- w172
      n202 = Divide(x=1000000.0, y=1000) -> (x/y=w180:dbl)
      n203 = node-c288(w180) -> (w184:T20)  [unwired: 3 in]
      n204 = timed-loop {
        timing: w184 -> [_]
        timing-out: [_] -> w183
        tunnel: w179 -> [w321]
        i -> [w322]
        stop <- w314 stop-if-true
        n205 = node-c288() -> ()  [unwired: 1 in, 1 out]
        n206 = global read "Global_vars.vi" "Mode test CL"() -> (w317:bool)
        n207 = Divide(x="PW test (0-100%)", y=100.0) -> (x/y=w323:dbl)
        n208 = global read "Global_vars.vi" "stop"() -> (w316:bool)
        n209 = Quotient & Remainder(x=w322, y=w321) -> (x-y*floor(x/y)=w319:dbl)  [unwired: 1 out]
        n210 = Multiply(x=w323, y=w321) -> (x*y=w318:dbl)
        n211 = Greater Or Equal?(x=w319, y=w318) -> (x >= y?=w320:bool)
        n212 = Compound Arithmetic op=OR(w317, w316, "stop test") -> (w314:bool)
        n213 = case shown="True" w320 {
          frame False {
            n214 = xnode "Digital output (1 sample) 5"("CH1 (A/DIO8 (Pin 27))"=TRUE) -> ()  [unwired: 1 in, 1 out]
          }
          frame True {
            n215 = xnode "Digital output (1 sample) 6"("CH1 (A/DIO8 (Pin 27))"=FALSE) -> ()  [unwired: 1 in, 1 out]
          }
        }
        n216 = node-c288() -> ()  [unwired: 1 in, 1 out]
      }
      n217 = node-c288(w183) -> ()  [unwired: 1 out]
      n218 = node-c288(w174) -> ()  [unwired: 1 out]
    }
    frame #2 {
      n219 = global write "Global_vars.vi" "stop"(FALSE ("stop")) -> ()
      n220 = xnode "Trigger 3"("C/DIO7 (DIO7)"=FALSE) -> ()  [unwired: 1 in, 1 out]
      n221 = xnode "Digital output (1 sample) 7"("CH1 (A/DIO8 (Pin 27))"=FALSE) -> ()  [unwired: 1 in, 1 out]
    }
  }
